vi "rollingAverage.vi"(8 "No Avg":i32, 10 "New Element":dbl, 11 "Rolling Array":dbl[](array[numeric])) -> (0 "standard deviation":dbl format="%0.2f", 1 "mean":dbl format="%0.2f", 3 "New Array":dbl[](array[numeric]))   [LabVIEW 2011]
uses:
  <vilib>/Analysis/NI_AALBase.lvlib
panel:
  # "Rolling Average"
  # "Al Fischer - 2016"
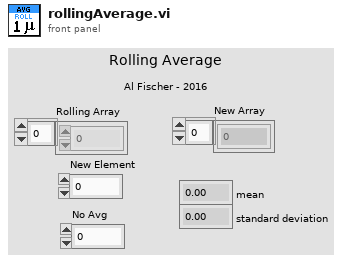
[diagram p1: front panel]
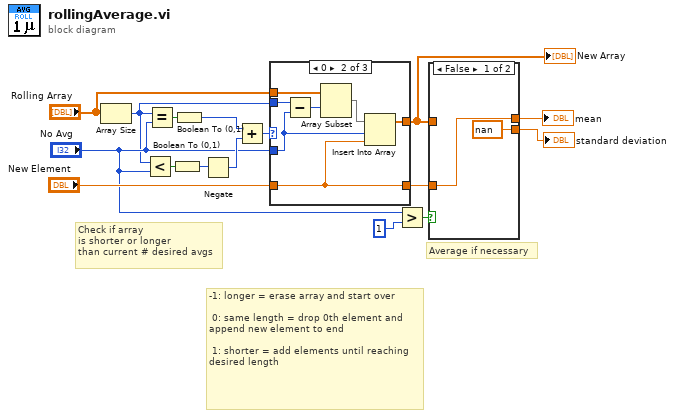
[diagram p0: block diagram]
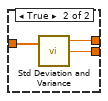
[diagram p2: hidden frame]
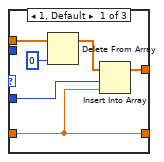
[diagram p3: hidden frame]
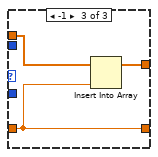
[diagram p4: hidden frame]
diagram:
  # "Average if necessary"
  # "-1: longer = erase array and start over\n\n 0: same length = drop 0th element and append new element to end\n\n 1: shorter = add elements until reaching desired length"
  # "Check if array\nis shorter or longer\nthan current # desired avgs"
  n1 = Array Size(array="Rolling Array") -> (size(s)=w1:i32)
  n2 = Less?(x=w1, y="No Avg") -> (x < y?=w10:bool)
  n3 = Equal?(x=w1, y="No Avg") -> (x = y?=w11:bool)
  n4 = Boolean To (0,1)(Boolean=w10) -> (0, 1=w7:i16)
  n5 = Boolean To (0,1)(Boolean=w11) -> (0, 1=w9:i16)
  n6 = Negate(x=w7) -> (-x=w6:i16)
  n7 = Add(x=w9, y=w6) -> (x+y=w8:i16)
  n8 = case shown="0" w8 {
    tunnel: "No Avg" -> [w18 w26 _]
    tunnel: [w22 w29 w31] -> w16
    tunnel: "Rolling Array" -> [w20 w27 w32]
    tunnel: "New Element" -> [w17 w28 w30]
    tunnel: [w17 w28 w30] -> w2
    tunnel: w1 -> [_ w25 _]
    frame 1, Default {
      n9 = Delete From Array(array=w20, index=0) -> (array with subset deleted=w19:dbl[])  [unwired: 1 in, 1 out]
      n10 = Insert Into Array(array=w19, index=w18, new element=w17) -> (w22:dbl[])
    }
    frame 0 {
      n11 = Subtract(x=w25, y=w26) -> (x-y=w23:i32)
      n12 = Array Subset(array=w27, index=w23) -> (w24:dbl[])  [unwired: 1 in]
      n13 = Insert Into Array(array=w24, index=w26, new element=w28) -> (w29:dbl[])
    }
    frame -1 {
      n14 = Insert Into Array(array=w32, new element=w30) -> (w31:dbl[])  [unwired: 1 in]
    }
  }
  "New Array" <- w16
  n15 = Greater?(x="No Avg", y=1) -> (0:w5:bool)
  n16 = case shown="False" w5 {
    tunnel: w16 -> [_ w37]
    tunnel: [nan ("standard deviation") w36] -> w13
    tunnel: [w34 w35] -> w12
    tunnel: w2 -> [w34 _]
    frame False {
    }
    frame True {
      n17 = call <vilib>:"Std Deviation and Variance.vi"("X"=w37) -> ("mean"=w35:dbl, "standard deviation"=w36:dbl)  [unwired: 1 in, 1 out]
    }
  }
  "mean" <- w12
  "standard deviation" <- w13
